vi "结束模块.vi"(11 "模块模板.i":refnum<class "模块模板.lvclass">) -> (3 "模块模板.o":refnum<class "模块模板.lvclass">)   [LabVIEW 2017, in "模块模板.lvlib" / "模块模板.lvclass"]
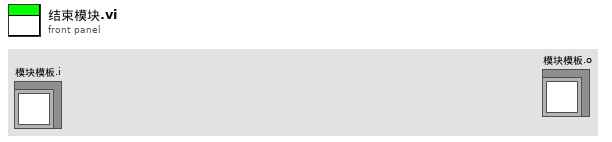
[diagram p1: front panel]
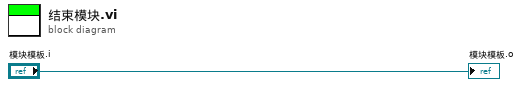
[diagram p0: block diagram]
diagram:
  "模块模板.o" <- "模块模板.i"
